vi "Modbus Serial Slave Example.vi"() -> ()   [LabVIEW 2013]
doc: "An example of the modbus master functionality."
uses:
  Network Protocol/Network Slave/daemon status.ctl
  Network Protocol/Network Slave/TCP/Connection.ctl
  API/Slave/Modbus Slave.lvclass
  Data Model/Identification Parameters.ctl
  API/Wrapper/Create Serial Slave.vi
  API/Wrapper/API Main.lvlib
  Data Model/Device Data Model.lvclass
  Network Protocol/Network Slave/Network Slave.lvclass
  Network Protocol/Network Slave/TCP/TCP Slave.lvclass
panel:
  in  "serial type":enum16{"RTU", "ASCII"}(ring)
  in  "Serial Resource":refnum<visa-resource-name>
  out "TCP Connection List":T1[](array[typedef])
  out "TCP Connection Count":u32
  out "Daemon Error":errorcluster
  out "Daemon Status":T2
  in  "Stop Button":bool
  in  "Fetch Holding Registers":bool
  in  "Fetch Coils":bool
  in  "Set Discrete Inputs":bool
  in  "Set Input Registers":bool
  in  "Set Basic Objects":bool
  in  "Basic Objects":string[](array[string])=["National Instruments", "42", "1.0.0"]
  out "Status":string
  out "Holding Registers":u16[](array[numeric])
  in  "Input Registers":u16[](array[numeric])=[0, 0, 0, 0, 0, 0, 0, 0]
  out "Coils":bool[](array[boolean])
  in  "Discrete Inputs":bool[](array[boolean])
  # "Holding Registers are the integer outputs of a modbus device. This example allows you to read the first 8 outputs."
  # "Coils are the boolean outputs of a modbus device. This example allows you to read the first 8 outputs."
  # "Modbus devices can also store objects in their memory, which are variable length strings. This example sets the basic level of objects."
  # "Discrete inputs are the boolean inputs of a modbus device. This example allows you to set the first 8 inputs."
  # "Input Registers are the integer inputs of a modbus device. This example allows you to set the first 8 inputs."
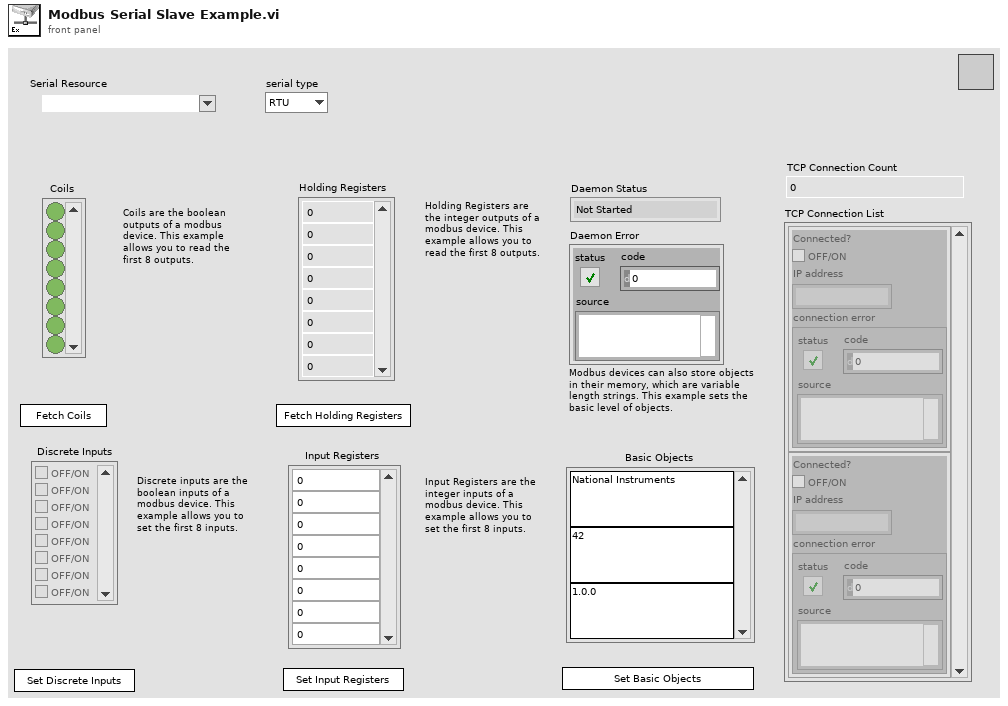
[diagram p1: front panel]
types:
  T1 = typedef "TCP Slave.lvclass/Connection.ctl" = cluster{"Connected?":bool, "IP address":string, "connection error":errorcluster}
  T2 = typedef "Network Slave.lvclass/daemon status.ctl" = enum16{"Not Started", "Running", "Error", "Stopped"}
  T3 = typedef "Device Data Model.lvclass/Identification Parameters.ctl" = cluster{"Object ID":u8, "Value":string}
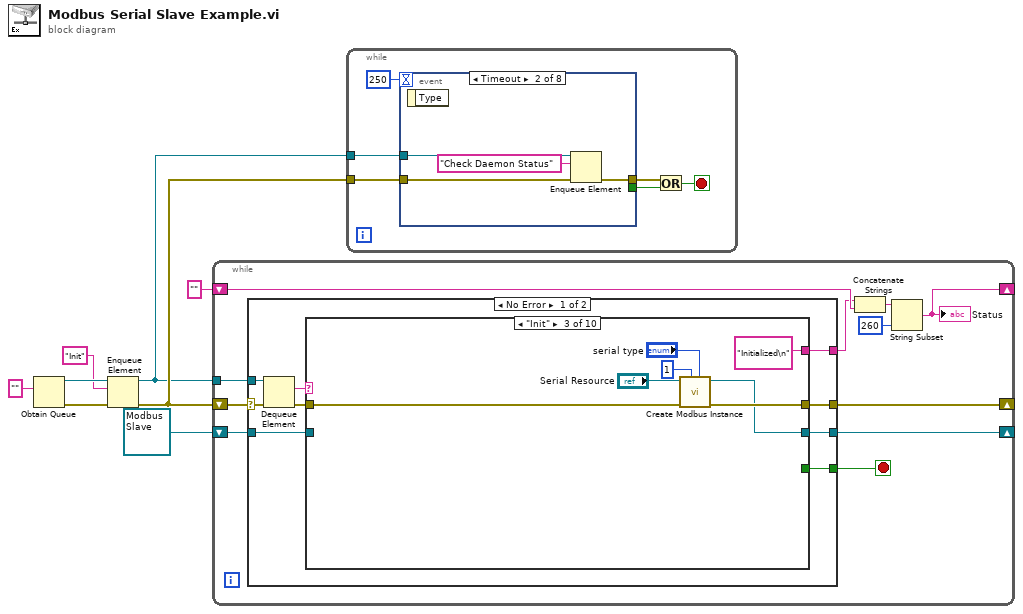
[diagram p0: block diagram]
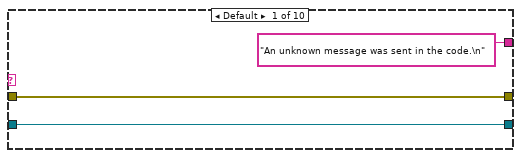
[diagram p2: hidden frame]
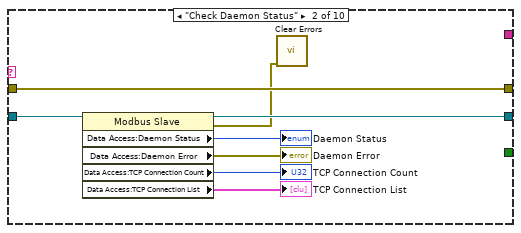
[diagram p3: hidden frame]
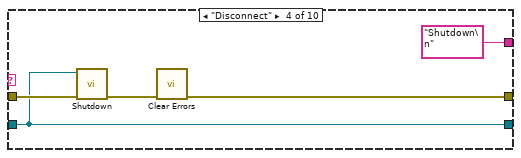
[diagram p4: hidden frame]
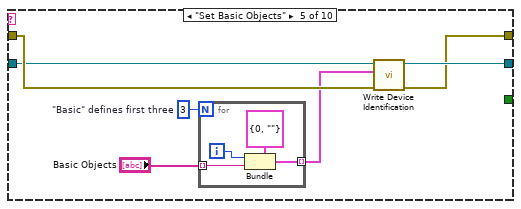
[diagram p5: hidden frame]
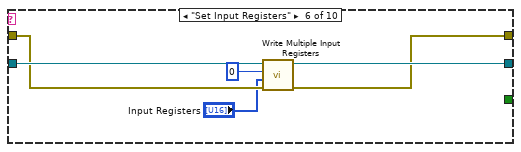
[diagram p6: hidden frame]
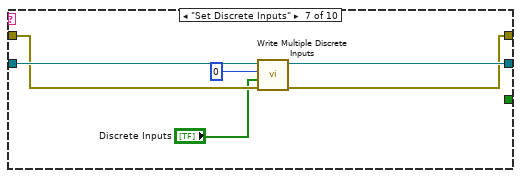
[diagram p7: hidden frame]
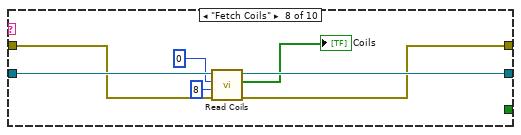
[diagram p8: hidden frame]
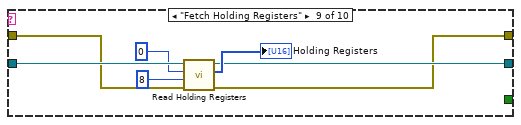
[diagram p9: hidden frame]
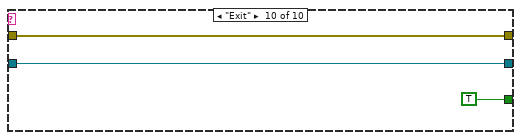
[diagram p10: hidden frame]
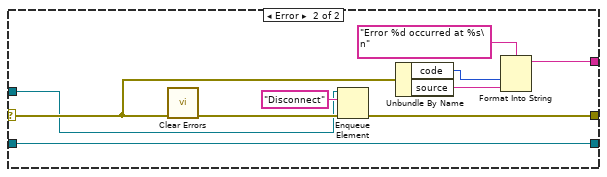
[diagram p11: hidden frame]
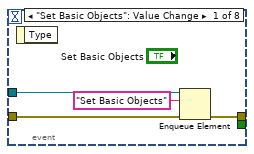
[diagram p12: hidden frame]
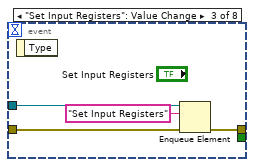
[diagram p13: hidden frame]
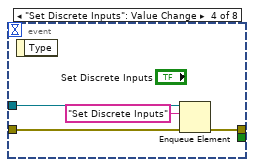
[diagram p14: hidden frame]
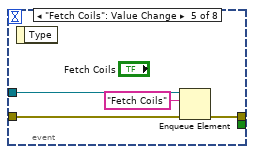
[diagram p15: hidden frame]
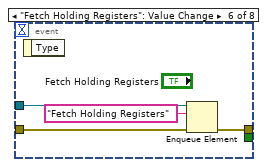
[diagram p16: hidden frame]
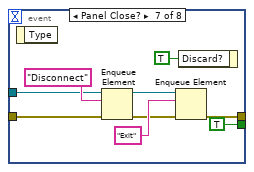
[diagram p17: hidden frame]
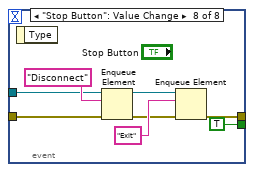
[diagram p18: hidden frame]
diagram:
  n1 = Obtain Queue(element data type="") -> (queue out=w4:refnum<queue>, error out=w8:errorcluster)  [unwired: 4 in, 1 out]
  n2 = Enqueue Element(queue=w4, element="Init", error in (no error)=w8) -> (queue out=w3:refnum<queue>, error out=w5:errorcluster)  [unwired: 1 in, 1 out]
  n3 = while {
    shift-right: [w9] -> _
    shift-left: refnum<class "Modbus Slave.lvclass"> refnum ("Modbus Slave") -> [w12]
    tunnel: w3 -> [w19]
    shift-right: [w10] -> _
    shift-left: w5 -> [w18]
    shift-right: [w17] -> _
    shift-left: "" ("Status") -> [w14]
    stop <- w11 stop-if-true
    n4 = case shown="No Error" w18 {
      selector: w18 -> [w27 w99]
      tunnel: w19 -> [w28 w93]
      tunnel: [w24 w100] -> w10
      tunnel: [w21 w96] -> w13
      tunnel: [w23 w92] -> w9
      tunnel: w12 -> [w22 w92]
      tunnel: [w20 _] -> w11
      frame No Error {
        n5 = Dequeue Element(queue=w28, error in (no error)=w27) -> (element=w25:string, error out=w26:errorcluster)  [unwired: 1 in, 2 out]
        n6 = case shown="\"Init\"" w25 {
          tunnel: w26 -> [w31 w39 w46 w51 w58 w65 w71 w78 w87 w91]
          tunnel: [w31 w39 w45 w47 w53 w66 w72 w76 w84 w91] -> w24
          tunnel: [w30 w37 w44 w49 w57 w67 w73 w77 w85 w90] -> w23
          tunnel: w22 -> [w30 w38 _ w49 w56 w68 w74 w81 w88 w90]
          tunnel: ["An unknown message was sent in the code.\n" _ "Initialized\n" "Shutdown\n" _ _ _ _ _ _] -> w21
          tunnel: [_ _ _ _ _ _ _ _ _ TRUE] -> w20
          frame Default {
          }
          frame "Check Daemon Status" {
            n7 = property class="Modbus Slave"(reference=w38) -> (reference out=w37:refnum<class "Modbus Slave.lvclass">, error out=w36:errorcluster, "Data Access:Daemon Status"=→"Daemon Status":T2, "Data Access:Daemon Error"=→"Daemon Error":errorcluster, "Data Access:TCP Connection Count"=→"TCP Connection Count":u32, "Data Access:TCP Connection List"=→"TCP Connection List":T1[])  [unwired: 1 in]
            n8 = call <vilib>:"Clear Errors.vi"("error in (no error)"=w36) -> ()  [unwired: 6 in, 1 out]
          }
          frame "Init" {
            n9 = call-poly "Create Modbus Instance.vi"("serial type"="serial type", "unit ID"=u8 1, "error in"=w46, "VISA resource name"="Serial Resource") -> ("error out"=w45:errorcluster, "serial slave instance"=w44:refnum<class "Modbus Slave.lvclass">)  [unwired: 6 in]
          }
          frame "Disconnect" {
            n10 = call-dynamic "Shutdown.vi"("error in"=w51, "Modbus slave in"=w49) -> ("error out"=w50:errorcluster)  [unwired: 9 in]
            n11 = call <vilib>:"Clear Errors.vi"("error in (no error)"=w50) -> ("error out"=w47:errorcluster)  [unwired: 6 in]
          }
          frame "Set Basic Objects" {
            w52 = 3  # "Basic" defines first three
            n12 = for {
              N: w52 -> [_]
              tunnel: "Basic Objects" -> [w60] mode=indexing
              tunnel: [w59] -> w54 mode=indexing
              i -> [w61]
              n13 = Bundle(cluster=T3 {"Object ID"=0, "Value"=""} ("Parameters"), "Object ID"=w61, "Value"=w60) -> (w59:T3)
            }
            n14 = call-dynamic "Write Device Identification.vi"("error in"=w58, "objects"=w54, "Modbus slave in"=w56) -> ("error out"=w53:errorcluster, "Modbus slave out"=w57:refnum<class "Modbus Slave.lvclass">)  [unwired: 7 in]
          }
          frame "Set Input Registers" {
            n15 = call-dynamic "Write Multiple Input Registers.vi"("error in"=w65, "input registers to write"="Input Registers", "starting address"=u16 0, "Modbus slave in"=w68) -> ("error out"=w66:errorcluster, "Modbus slave out"=w67:refnum<class "Modbus Slave.lvclass">)  [unwired: 6 in]
          }
          frame "Set Discrete Inputs" {
            n16 = call-dynamic "Write Multiple Discrete Inputs.vi"("error in"=w71, "discrete inputs to write"="Discrete Inputs", "starting address"=u16 0, "Modbus slave in"=w74) -> ("error out"=w72:errorcluster, "Modbus slave out"=w73:refnum<class "Modbus Slave.lvclass">)  [unwired: 6 in]
          }
          frame "Fetch Coils" {
            n17 = call-dynamic "Read Coils.vi"("error in"=w78, "number of inputs"=u16 8 ("number of coils"), "starting address"=u16 0, "Modbus slave in"=w81) -> ("error out"=w76:errorcluster, "coils"=→"Coils":bool[], "Modbus slave out"=w77:refnum<class "Modbus Slave.lvclass">)  [unwired: 5 in]
          }
          frame "Fetch Holding Registers" {
            n18 = call-dynamic "Read Holding Registers.vi"("error in"=w87, "number of inputs"=u16 8 ("number of registers"), "starting address"=u16 0, "Modbus slave in"=w88) -> ("error out"=w84:errorcluster, "register values"=→"Holding Registers":u16[], "Modbus slave out"=w85:refnum<class "Modbus Slave.lvclass">)  [unwired: 5 in]
          }
          frame "Exit" {
          }
        }
      }
      frame Error {
        n19 = call <vilib>:"Clear Errors.vi"("error in (no error)"=w99) -> ("error out"=w101:errorcluster)  [unwired: 6 in]
        n20 = Enqueue Element(queue=w93, element="Disconnect", error in (no error)=w101) -> (error out=w100:errorcluster)  [unwired: 1 in, 2 out]
        n21 = Unbundle By Name(w99) -> ("code"=w98:i32, "source"=w97:string)
        n22 = Format Into String(format string="Error %d occurred at %s\n", w98, w97) -> (resulting string=w96:string)  [unwired: 2 in, 1 out]
      }
    }
    n23 = Concatenate Strings(w13, w14) -> (w15:string)
    n24 = String Subset(string=w15, length (rest)=260 ("length (rest)")) -> (substring=w17:string)  [unwired: 1 in]
    "Status" <- w17
  }
  n25 = while {
    tunnel: w5 -> [w107]
    tunnel: w3 -> [w106]
    stop <- w103 stop-if-true
    n26 = event shown="[1] Timeout" {
      selector: _ -> [_ _ _ _ _ _ _ _]
      dyn-events: _ -> [_ _ _ _ _ _ _ _]
      timeout: 250 -> [_ _ _ _ _ _ _ _]
      tunnel: w107 -> [w111 w115 w119 w123 w127 w131 w137 w146]
      tunnel: [w110 w114 w118 w122 w126 w130 w132 w141] -> w105
      tunnel: w106 -> [w109 w113 w117 w121 w125 w129 w134 w143]
      tunnel: [_ _ _ _ _ _ TRUE ("Discard?") TRUE ("Discard?")] -> w104
      event "Set Basic Objects": Value Change {
        n27 = event-data() -> ()  [unwired: 1 in, 1 out]
        n28 = Enqueue Element(queue=w109, element="Set Basic Objects", error in (no error)=w111) -> (error out=w110:errorcluster)  [unwired: 1 in, 2 out]
      }
      event Timeout {
        n29 = event-data() -> ()  [unwired: 1 in, 1 out]
        n30 = Enqueue Element(queue=w113, element="Check Daemon Status", error in (no error)=w115) -> (error out=w114:errorcluster)  [unwired: 1 in, 2 out]
      }
      event "Set Input Registers": Value Change {
        n31 = event-data() -> ()  [unwired: 1 in, 1 out]
        n32 = Enqueue Element(queue=w117, element="Set Input Registers", error in (no error)=w119) -> (error out=w118:errorcluster)  [unwired: 1 in, 2 out]
      }
      event "Set Discrete Inputs": Value Change {
        n33 = event-data() -> ()  [unwired: 1 in, 1 out]
        n34 = Enqueue Element(queue=w121, element="Set Discrete Inputs", error in (no error)=w123) -> (error out=w122:errorcluster)  [unwired: 1 in, 2 out]
      }
      event "Fetch Coils": Value Change {
        n35 = event-data() -> ()  [unwired: 1 in, 1 out]
        n36 = Enqueue Element(queue=w125, element="Fetch Coils", error in (no error)=w127) -> (error out=w126:errorcluster)  [unwired: 1 in, 2 out]
      }
      event "Fetch Holding Registers": Value Change {
        n37 = event-data() -> ()  [unwired: 1 in, 1 out]
        n38 = Enqueue Element(queue=w129, element="Fetch Holding Registers", error in (no error)=w131) -> (error out=w130:errorcluster)  [unwired: 1 in, 2 out]
      }
      event Panel Close? {
        n39 = event-data() -> ()  [unwired: 1 in, 1 out]
        n40 = Enqueue Element(queue=w134, element="Disconnect", error in (no error)=w137) -> (queue out=w135:refnum<queue>, error out=w133:errorcluster)  [unwired: 1 in, 1 out]
        n41 = Enqueue Element(queue=w135, element="Exit", error in (no error)=w133) -> (error out=w132:errorcluster)  [unwired: 1 in, 2 out]
        n42 = event-data("Discard?"=TRUE) -> ()  [unwired: 1 in, 1 out]
      }
      event "Stop Button": Value Change {
        n43 = event-data() -> ()  [unwired: 1 in, 1 out]
        n44 = Enqueue Element(queue=w143, element="Disconnect", error in (no error)=w146) -> (queue out=w144:refnum<queue>, error out=w142:errorcluster)  [unwired: 1 in, 1 out]
        n45 = Enqueue Element(queue=w144, element="Exit", error in (no error)=w142) -> (error out=w141:errorcluster)  [unwired: 1 in, 2 out]
      }
    }
    n46 = Or(x=w105, y=w104) -> (x .or. y?=w103:bool)
  }
